vi "JsonToAttrMap.vi"(7 "Type and Defaults":variant, 8 "error in (no error)":errorcluster, 11 "Json":string) -> (0 "error out":errorcluster, 3 "AttrMap":T1)   [LabVIEW 2019]
uses:
  Typedef/Def-AttrMap.ctl
  <vilib>/Utility/error.llb/Clear Errors.vi
  Json/Remove Comments.vi
  <userlib>/NEVSTOP-Programming-Palette/Configuration/Ini/TextToLines.vi
  <userlib>/_OpenG.lib/array/array.llb/Filter 1D Array__ogtk.vi
  <userlib>/_OpenG.lib/array/array.llb/Filter 1D Array (U8)__ogtk.vi
  <userlib>/NEVSTOP-Programming-Palette/Configuration/Ini/LinesToText.vi
  <vilib>/Utility/error.llb/Error Cluster From Error Code.vi
  <vilib>/addons/_JKI.lib/Serialization/JSON/JKI JSON Serialization.lvlib
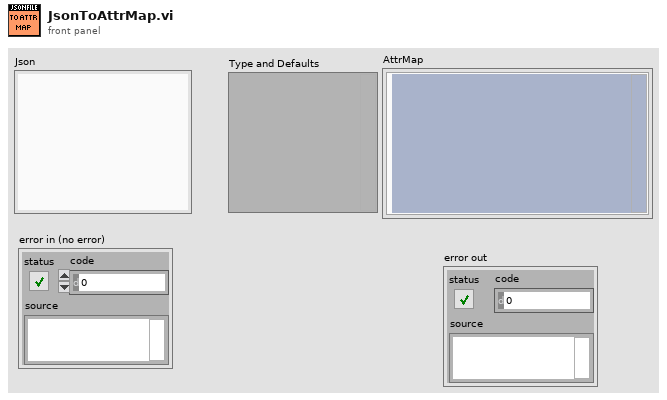
[diagram p1: front panel]
types:
  T1 = typedef "Def-AttrMap.ctl" = cluster{"Map":variant}
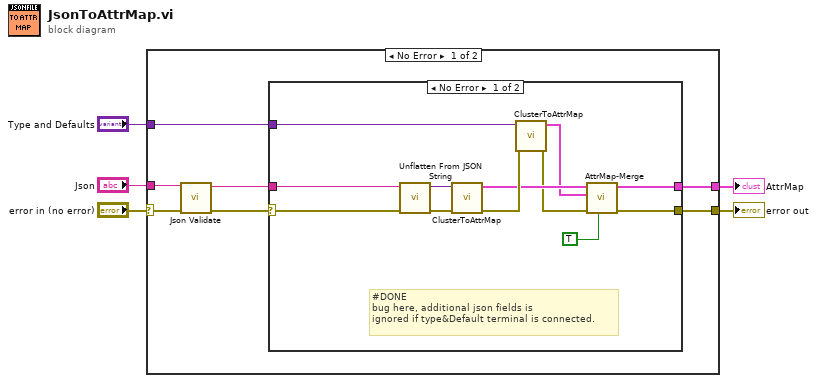
[diagram p0: block diagram]
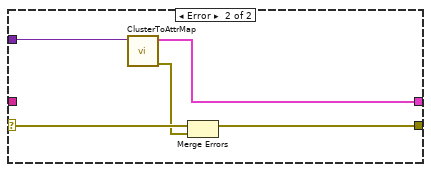
[diagram p2: hidden frame]
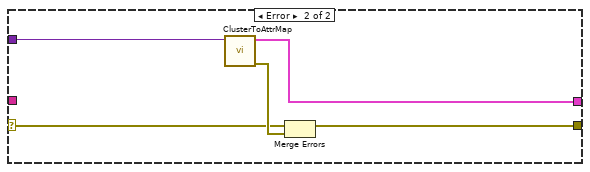
[diagram p3: hidden frame]
diagram:
  n1 = case shown="No Error" "error in (no error)" {
    selector: "error in (no error)" -> [w11 w31]
    tunnel: "Json" -> [w12 _]
    tunnel: "Type and Defaults" -> [w9 w33]
    tunnel: [w8 w30] -> w2
    tunnel: [w7 w32] -> w1
    frame No Error {
      n2 = call "Json Validate.vi"("error in (no error)"=w11, "String"=w12) -> ("error out"=w10:errorcluster, "Json without comments"=w6:string)  [unwired: 6 in, 2 out]
      n3 = case shown="No Error" w10 {
        selector: w10 -> [w21 w29]
        tunnel: w6 -> [w24 _]
        tunnel: w9 -> [w20 w28]
        tunnel: [w15 w27] -> w8
        tunnel: [w17 w26] -> w7
        frame No Error {
          # "#DONE\nbug here, additional json fields is\nignored if type&Default terminal is connected."
          n4 = call <vilib>:"Unflatten From JSON String.vi"("error in (no error)"=w21, "JSON String"=w24) -> ("error out"=w22:errorcluster, "Variant"=w23:variant)  [unwired: 8 in]
          n5 = call "ClusterToAttrMap.vi"("error in (no error)"=w22, "data"=w23) -> ("error out"=w19:errorcluster, "AttrMap"=w18:T1)  [unwired: 8 in]
          n6 = call "ClusterToAttrMap.vi"("error in (no error)"=w19, "data"=w20) -> ("error out"=w16:errorcluster, "AttrMap"=w14:T1)  [unwired: 8 in]
          n7 = call "AttrMap-Merge.vi"("If exist? Skip(T)/Overwrite(F)"=TRUE, "error in (no error)"=w16, "AttrMap B"=w14, "AttrMap A"=w18) -> ("error out"=w15:errorcluster, "AttrMap A after B->A"=w17:T1)  [unwired: 6 in]
        }
        frame Error {
          n8 = call "ClusterToAttrMap.vi"("data"=w28) -> ("error out"=w25:errorcluster, "AttrMap"=w26:T1)  [unwired: 9 in]
          n9 = Merge Errors(w29, w25) -> (w27:errorcluster)
        }
      }
    }
    frame Error {
      n10 = call "ClusterToAttrMap.vi"("data"=w33) -> ("error out"=w34:errorcluster, "AttrMap"=w32:T1)  [unwired: 9 in]
      n11 = Merge Errors(w31, w34) -> (w30:errorcluster)
    }
  }
  "error out" <- w2
  "AttrMap" <- w1
